vi "Panic.vi"(11 "message (\"\")":string) -> ()   [LabVIEW 2018, in "Utilities.lvlib"]
uses:
  Utilities.lvlib
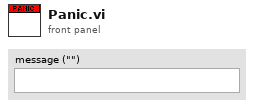
[diagram p1: front panel]
types:
  T1 = enum32{"invalid app kind", "Development System", "Run Time System", "Student Edition", "Embedded LabVIEW", "Evaluation", "Custom"}
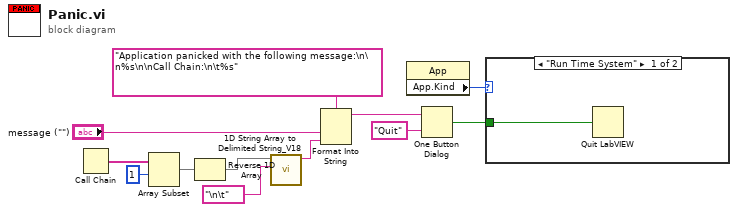
[diagram p0: block diagram]
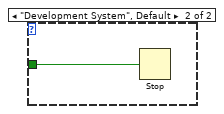
[diagram p2: hidden frame]
diagram:
  n1 = Call Chain() -> (call chain=w5:string[])
  n2 = Array Subset(array=w5, index=1) -> (w4:string[])  [unwired: 1 in]
  n3 = Reverse 1D Array(array=w4) -> (reversed array=w3:string[])
  n4 = call "1D String Array to Delimited String_V18.vi"("delimiter"="\n\t", "string array"=w3) -> ("delimited string"=w1:string)  [unwired: 9 in]
  n5 = Format Into String(format string="Application panicked with the following message:\n\n%s\n\nCall Chain:\n\t%s", "message (\"\")", w1) -> (resulting string=w7:string)  [unwired: 2 in, 1 out]
  n6 = property class="App"() -> ("App.Kind"=w12:T1)  [unwired: 2 in, 2 out]
  n7 = One Button Dialog(message=w7, button name ("OK")="Quit") -> (true=w11:bool)
  n8 = case shown="\"Run Time System\"" w12 {
    tunnel: w11 -> [w13 w14]
    frame "Run Time System" {
      n9 = Quit LabVIEW(quit? (T)=w13) -> ()
    }
    frame "Development System", Default {
      n10 = Stop(stop? (T)=w14) -> ()
    }
  }
